vi "Telemetry Name Reader.vi"(11 "Digital Channels":path=path "C:/Users/david/OneDrive/Desktop/New Data/Digital Data.txt") -> (3 "Digital Signal Names":string[](array[string]))   [LabVIEW 2021]
uses:
  <vilib>/Utility/file.llb/Read Delimited Spreadsheet (string).vi
panel:
  out "Digital Command Names":string[](array[string])
  out "Aux2 Analog Names":string[](array[string])
  out "size(s) 4":i32
  out "Aux1 Analog Names":string[](array[string])
  out "size(s) 3":i32
  out "Exec Analog Names":string[](array[string])
  out "size(s) 2":i32
  in  "Aux2 Analog Channels":path=path "C:/Users/david/OneDrive/Desktop/New Data/Aux 2 Analog Input Data.txt"
  in  "Aux1 Analog Channels":path=path "C:/Users/david/OneDrive/Desktop/New Data/Aux1 Analog Input Data.txt"
  in  "Exec Analog Channels":path=path "C:/Users/david/OneDrive/Desktop/New Data/Exec Analog Input Data.txt"
  out "size(s)":i32
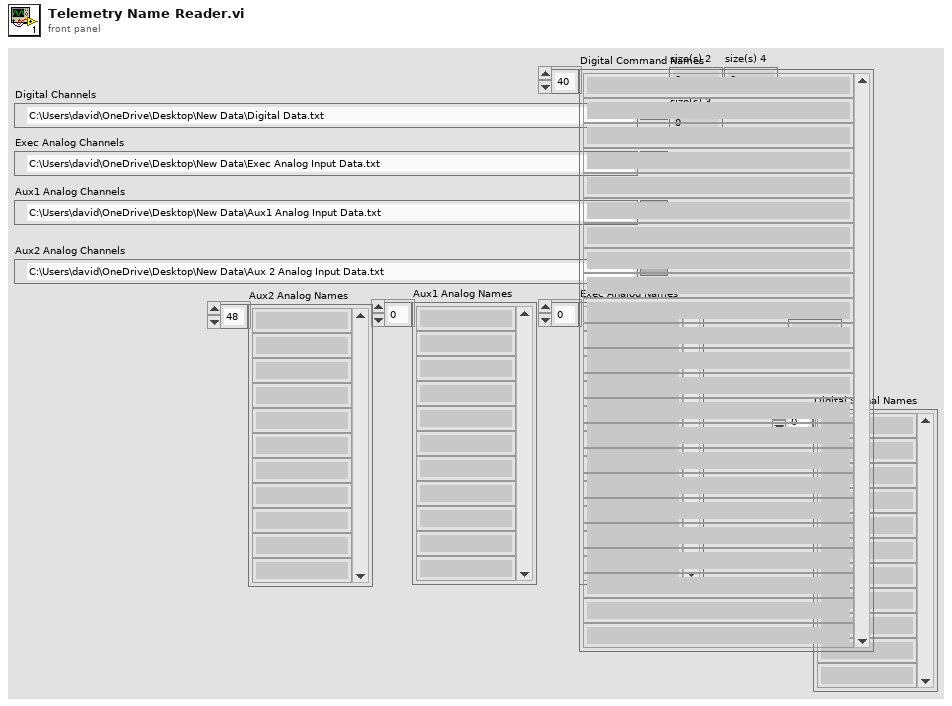
[diagram p1: front panel]
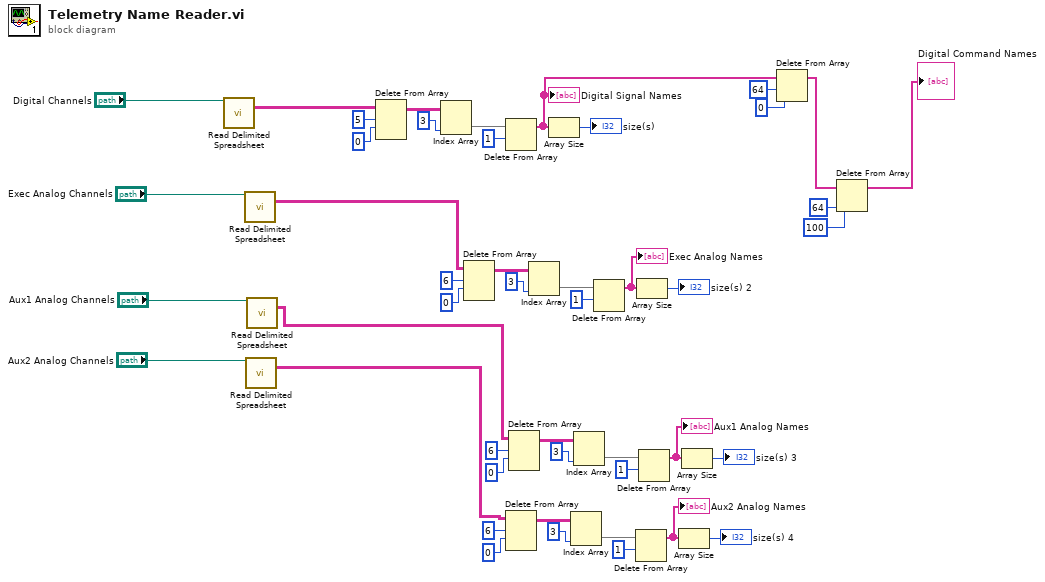
[diagram p0: block diagram]
diagram:
  n1 = call-poly <vilib>:"Read Delimited Spreadsheet.vi"("file path (dialog if empty)"="Digital Channels") -> ("all rows"=w45:string[][])  [unwired: 9 in, 5 out]
  n2 = call-poly <vilib>:"Read Delimited Spreadsheet.vi"("file path (dialog if empty)"="Exec Analog Channels") -> ("all rows"=w10:string[][])  [unwired: 9 in, 5 out]
  n3 = call-poly <vilib>:"Read Delimited Spreadsheet.vi"("file path (dialog if empty)"="Aux2 Analog Channels") -> ("all rows"=w8:string[][])  [unwired: 9 in, 5 out]
  n4 = call-poly <vilib>:"Read Delimited Spreadsheet.vi"("file path (dialog if empty)"="Aux1 Analog Channels") -> ("all rows"=w9:string[][])  [unwired: 9 in, 5 out]
  n5 = Delete From Array(array=w45, length=5, index (row)=0) -> (array with subset deleted=w42:string[][])  [unwired: 1 in, 1 out]
  n6 = Index Array(array=w42, index (col)=3 ("disabled index (col)")) -> (element=w39:string[])  [unwired: 1 in]
  n7 = Delete From Array(array=w10, length=6, index (row)=0) -> (array with subset deleted=w29:string[][])  [unwired: 1 in, 1 out]
  n8 = Delete From Array(array=w39, length=1) -> (array with subset deleted=w1:string[])  [unwired: 1 in, 1 out]
  "Digital Signal Names" <- w1
  n9 = Delete From Array(array=w8, length=6, index (row)=0) -> (array with subset deleted=w13:string[][])  [unwired: 1 in, 1 out]
  n10 = Delete From Array(array=w9, length=6, index (row)=0) -> (array with subset deleted=w24:string[][])  [unwired: 1 in, 1 out]
  n11 = Index Array(array=w29, index (col)=3 ("disabled index (col)")) -> (element=w32:string[])  [unwired: 1 in]
  n12 = Array Size(array=w1) -> (size(s)=→"size(s)":i32)
  n13 = Index Array(array=w13, index (col)=3 ("disabled index (col)")) -> (element=w16:string[])  [unwired: 1 in]
  n14 = Index Array(array=w24, index (col)=3 ("disabled index (col)")) -> (element=w21:string[])  [unwired: 1 in]
  n15 = Delete From Array(array=w32, length=1) -> (array with subset deleted=w33:string[])  [unwired: 1 in, 1 out]
  "Exec Analog Names" <- w33
  n16 = Delete From Array(array=w16, length=1) -> (array with subset deleted=w17:string[])  [unwired: 1 in, 1 out]
  "Aux2 Analog Names" <- w17
  n17 = Array Size(array=w33) -> (size(s)=→"size(s) 2":i32)
  n18 = Delete From Array(array=w21, length=1) -> (array with subset deleted=w20:string[])  [unwired: 1 in, 1 out]
  "Aux1 Analog Names" <- w20
  n19 = Array Size(array=w17) -> (size(s)=→"size(s) 4":i32)
  n20 = Array Size(array=w20) -> (size(s)=→"size(s) 3":i32)
  n21 = Delete From Array(array=w1, length=64, index=0) -> (array with subset deleted=w5:string[])  [unwired: 1 out]
  n22 = Delete From Array(array=w5, length=100, index=64) -> (array with subset deleted=→"Digital Command Names":string[])  [unwired: 1 out]
